vi "YKMW100 Write Com Register.vi"(0 "VISA session":refnum<visa-resource-name>="MW100", 5 "Channel":string="C001", 7 "Value":string="000", 11 "error in (no error)":errorcluster) -> (4 "dup VISA session":refnum<visa-resource-name>="MW100", 15 "error out":errorcluster)   [LabVIEW 2016]
panel:
  out "CMD":string
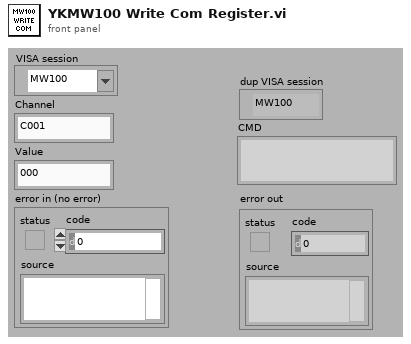
[diagram p1: front panel]
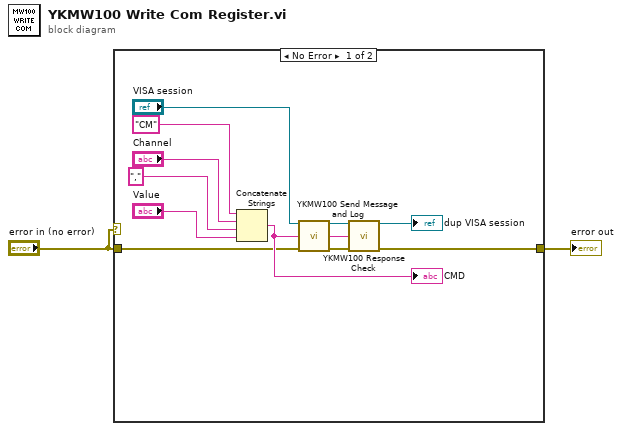
[diagram p0: block diagram]
diagram:
  n1 = case shown="No Error" "error in (no error)" {
    selector: "error in (no error)" -> [_ w15]
    tunnel: [w3 w15] -> w2
    tunnel: "error in (no error)" -> [w4 _]
    frame No Error {
      n2 = Concatenate Strings("CM" ("string"), "Channel", "," ("string"), "Value") -> (w5:string)
      "CMD" <- w5
      n3 = call "YKMW100 Send Message and Log.vi"("VISA session"="VISA session", "Send Message (\"\")"=w5, "error in (no error)"=w4) -> ("dup VISA session"=w14:refnum<visa-resource-name>, "Read Buffer"=w12:string, "error out"=w13:errorcluster)  [unwired: 10 in]
      n4 = call "YKMW100 Response Check.vi"("VISA session"=w14, "Message In (\"\")"=w12, "error in (no error)"=w13) -> ("dup VISA session"=→"dup VISA session":refnum<visa-resource-name>, "error out"=w3:errorcluster)  [unwired: 8 in, 3 out]
    }
    frame Error {
    }
  }
  "error out" <- w2
